vi "read_from_db.vi"(7 "condition":string, 9 "table":string, 11 "connection information":path) -> (3 "data":string[][](array[string]))   [LabVIEW 2017]
uses:
  <vilib>/addons/database/Connection.llb/DB Tools Open Connec (Path).vi
  <vilib>/addons/database/_DB Variant To Data/Database Variant To Data.xnode
  <vilib>/addons/database/NI_Database_API.lvlib
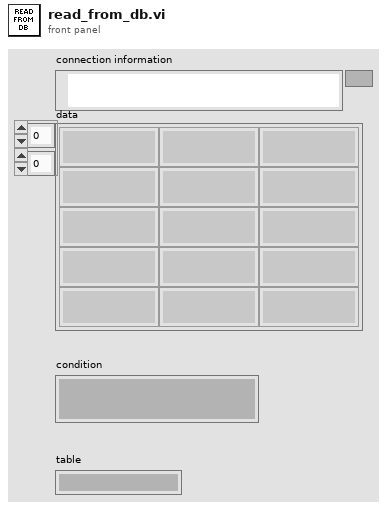
[diagram p1: front panel]
types:
  T1 = typedef "NI_Database_API.lvlib/Conn ObjectReference.ctl" = refnum<k1>
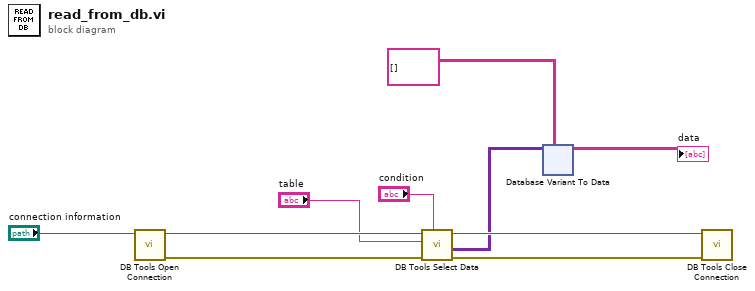
[diagram p0: block diagram]
diagram:
  n1 = call-poly <vilib>:"DB Tools Open Connection.vi"("connection information"="connection information") -> ("error out"=w9:errorcluster, "connection reference"=w10:T1)  [unwired: 7 in]
  n2 = call <vilib>:"DB Tools Select Data.vi"("condition"="condition", "error in (no error)"=w9, "table"="table", "connection reference"=w10) -> ("error out"=w7:errorcluster, "data"=w5:variant[][], "connection reference out"=w8:T1)  [unwired: 2 in]
  n3 = xnode "Database Variant To Data"("database variant"=w5, "type"=string[][] []) -> ("data"=→"data":string[][])  [unwired: 1 in, 1 out]
  n4 = call <vilib>:"DB Tools Close Connection.vi"("error in (no error)"=w7, "connection reference"=w8) -> ()  [unwired: 5 in, 1 out]
